vi "平面度.vi"(2 "Z":dbl[](array[numeric])=[76.1028438, 95.2953608, 114.4714072, 133.7959897, 152.7293809, 172.16341820000002, 66.5043349, 85.8245233, 104.86318860000002, 124.1722705, 143.1851144, 162.7298966, 61.8712851, 91.7690228, 111.0170432, 130.1167603, 149.37196840000001, 168.4774861, 187.7164273, 82.16492670000001, 101.4261197, 120.543452, 139.7336895, 158.8725655, 178.3698274, 82.2860118, 43.760144000000004, 43.728344, 43.976735999999995, 43.88023200000001, 44.00264, 43.968888, 24.709063999999998, 24.706424, 24.741704000000002, 24.824184000000002, 24.775544000000004, 24.845632000000002, 5.536616, 59.133488, 59.205760000000005, 59.216472, 59.23180000000001, 59.4576, 59.318304, 40.076744, 40.082808, 40.167384], 3 "Y":dbl[](array[numeric])=[84.03392269999999, 103.8371226, 81.29468150000001, 100.4252349, 119.7946411, 138.9026711, 157.9835411, 71.7289392, 91.02511039999999, 110.1892258, 129.4159159, 148.6512099, 100.2903467, 120.1801967, 96.9436818, 116.05569849999999, 135.3803877, 154.5082542, 173.6034899, 87.3906077, 106.64211039999999, 125.7939456, 144.9953381, 164.22002030000002, 44.403536, 44.219512, 25.29652, 25.307216, 25.329864, 25.417208, 25.390104, 6.1198559999999995, 6.1700479999999995, 6.197952000000001, 6.265904000000001, 6.299272, 49.562848, 49.565744, 40.664728000000004, 40.655392, 40.722648, 40.763424, 40.742984, 21.552992, 21.593224, 21.623056000000002, 21.687664, 21.735024000000003], 4 "X":dbl[](array[numeric])=[-21.99849438339363, -22.040277448755994, -22.00695671437586, -22.01434541657512, -21.986329148271935, -21.96213235076033, -21.940738941012977, -21.929642458923098, -21.89498672356566, -21.90856832311142, -21.884057999034457, -21.883311764692547, -21.84588856629861, -21.843707188106638, -21.715757587408998, -21.765079026013318, -21.77066598370853, -21.782598372453904, -21.775776519905722, -21.7897940876202, -21.783365005453096, -21.770305603359834, -21.759254769103705, -21.759031404220167, -21.75102086954063, -21.695065999869225, -21.750653875779278, -21.763772456326404, -21.79401962113512, -21.82854396443584, -21.801068240696907, -21.85672600592004, -21.87279533146989, -21.859192438198054, -21.888398314720497, -21.896856527913606, -21.91640738425516, -21.89663198955744, -21.92319142701181, -21.902006172480455, -21.90934696984737, -21.940179892141536, -21.9592704353829, -21.959077418017593, -21.94193604253543, -21.937335225540007, -21.898748915823067, -21.857716090298865]) -> (0 "x-y":dbl=192.37313427964241, 1 "£GZ":dbl[](array[numeric])=[-10.560458642860866, -4.938075893844172, 30.448806624908755, 34.896087707550976, 36.863098398112896, 39.744229747811005, -82.29576027139774, 5.293510449582058, 7.068262297732375, 11.805305230182086, 14.153696148943737, 18.301365826013495, -45.9534332519486, -32.05234453592051, -1.1132692631592676, 5.372342328233685, 9.498646647508167, 13.972636589025711, 17.600515881259895, -18.368617301668124, -14.822186865278198, -11.695556395140898, -8.427888703327511, -4.649617161165281, 110.07737400824467, 11.140228696658724, -9.297301946961475, -8.634234649352827, -6.7820979385247355, -5.097170747989111, -6.426347631754581, 11.909227644194182, -6.529045568816073, -7.2833388103169625, -5.736316933157266, -5.226955348242711, -38.768128015238595, -39.7606914492824, -50.53920848731955, 1.9291824314721566, 2.3413656123393096, 3.972757068648825, 5.028022170680501, 20.56440456859268, 19.473882568702365, -0.03818651649040561, -2.1526684278077255, -4.306047889620771])   [LabVIEW 2015]
uses:
  <vilib>/Analysis/7linalg.llb/Solve Linear Equations (single right hand).vi
  <vilib>/Analysis/baseanly.llb/Solve Linear Equations By Cholesky.vi
  <vilib>/Analysis/baseanly.llb/Real Matrix to Compact Array.vi
  <vilib>/Analysis/baseanly.llb/Real Compact Tri-Matrix Linear Eqs.vi
  <vilib>/Analysis/7linalg.llb/Solve Linear Eqs (General).vi
  <vilib>/Analysis/7linalg.llb/Solve Linear Eqs (Gen, single right hand).vi
  <vilib>/Analysis/NI_AALPro.lvlib
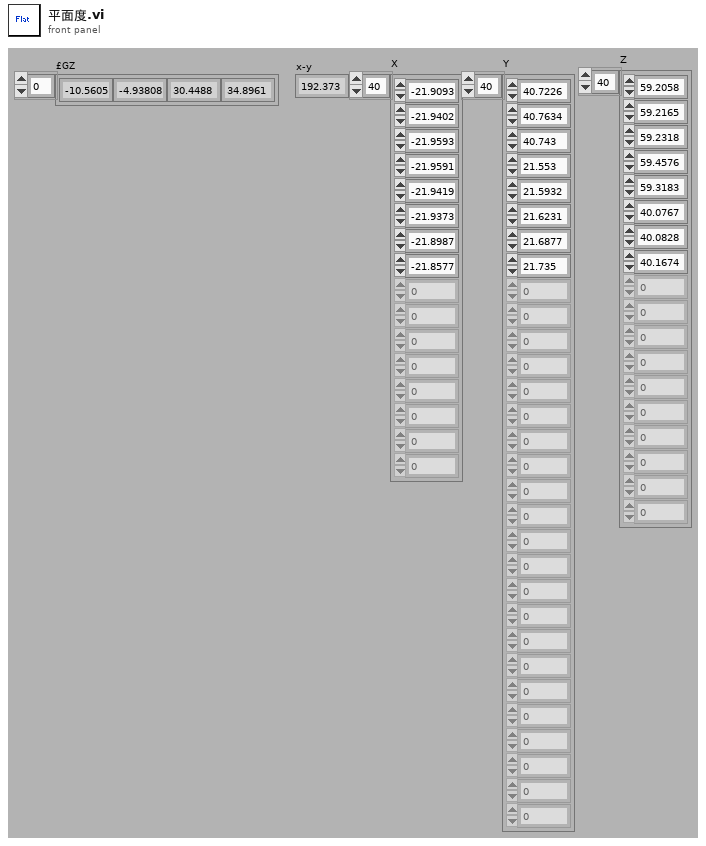
[diagram p1: front panel]
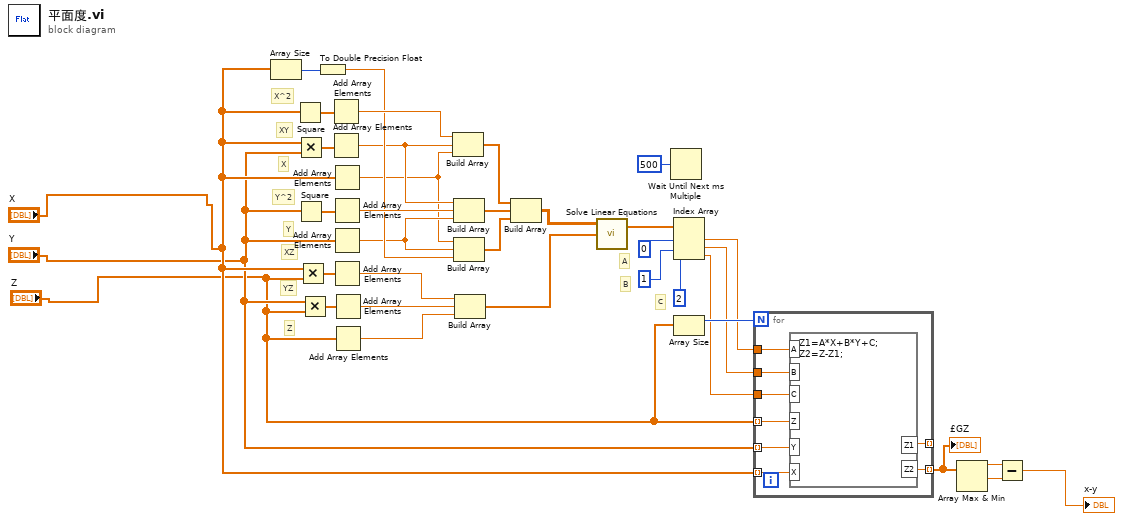
[diagram p0: block diagram]
diagram:
  # "C"
  # "B"
  # "A"
  # "Z"
  # "XZ"
  # "YZ"
  # "Y"
  # "Y^2"
  # "XY"
  # "X"
  # "X^2"
  n1 = Array Size(array="X") -> (size(s)=w25:i32)
  n2 = Square(x="X") -> (x^2=w36:dbl[])
  n3 = Multiply(x="X", y="Y") -> (x*y=w10:dbl[])
  n4 = Square(x="Y") -> (x^2=w35:dbl[])
  n5 = Multiply(x="X", y="Z") -> (x*y=w34:dbl[])
  n6 = Multiply(x="Y", y="Z") -> (x*y=w33:dbl[])
  n7 = To Double Precision Float(number=w25) -> (double precision float=w24:dbl)
  n8 = Add Array Elements(numeric array=w36) -> (sum=w32:dbl)
  n9 = Add Array Elements(numeric array=w10) -> (sum=w9:dbl)
  n10 = Add Array Elements(numeric array="X") -> (sum=w8:dbl)
  n11 = Add Array Elements(numeric array=w35) -> (sum=w31:dbl)
  n12 = Add Array Elements(numeric array="Y") -> (sum=w20:dbl)
  n13 = Add Array Elements(numeric array=w34) -> (sum=w30:dbl)
  n14 = Add Array Elements(numeric array=w33) -> (sum=w29:dbl)
  n15 = Add Array Elements(numeric array="Z") -> (sum=w19:dbl)
  n16 = Build Array(w32, w9, w8) -> (w28:dbl[])
  n17 = Build Array(w9, w31, w20) -> (w27:dbl[])
  n18 = Build Array(w8, w20, w24) -> (w26:dbl[])
  n19 = Build Array(w30, w29, w19) -> (w6:dbl[])
  n20 = Build Array(w28, w27, w26) -> (w7:dbl[][])
  n21 = call-poly <vilib>:"Solve Linear Equations.vi"("Known Vector"=w6, "Input Matrix"=w7) -> ("Solution Vector"=w14:dbl[])  [unwired: 1 in, 1 out]
  n22 = Wait Until Next ms Multiple(millisecond multiple=u32 500) -> ()  [unwired: 1 out]
  n23 = Index Array(array=w14, index #1=0 ("index"), index #2=1 ("index"), index #3=2 ("index")) -> (element #1=w13:dbl, element #2=w12:dbl, element #3=w11:dbl)
  n24 = Array Size(array="Z") -> (size(s)=w17:i32)
  n25 = for {
    N: w17 -> [_]
    tunnel: "X" -> [w44] mode=indexing
    tunnel: "Y" -> [w43] mode=indexing
    tunnel: "Z" -> [w42] mode=indexing
    tunnel: w11 -> [w41]
    tunnel: w12 -> [w40]
    tunnel: w13 -> [w39]
    tunnel: [w38] -> w2 mode=indexing
    tunnel: [w37] -> _ mode=indexing
    n26 = formula code="Z1=A*X+B*Y+C;\nZ2=Z-Z1;"("Z"=w42, "Y"=w43, "X"=w44, "A"=w39, "B"=w40, "C"=w41) -> ("Z2"=w38:dbl, "Z1"=w37:dbl)
  }
  "£GZ" <- w2
  n27 = Array Max & Min(array=w2) -> (max value=w16:dbl, min value=w15:dbl)  [unwired: 2 out]
  n28 = Subtract(x=w16, y=w15) -> (x-y=→"x-y":dbl)
